vi "get-locking.vi"() -> (0 "error out":errorcluster, 3 "locking":u8)   [LabVIEW 2014]
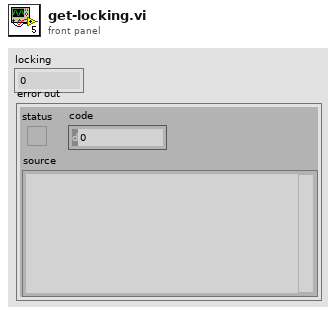
[diagram p1: front panel]
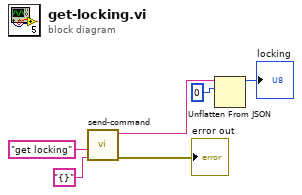
[diagram p0: block diagram]
diagram:
  n1 = call "send-command.vi"("parameters"="{}", "command"="get locking") -> ("error out"=→"error out":errorcluster, "output"=w3:string)  [unwired: 8 in]
  n2 = Unflatten From JSON(JSON string=w3, type and defaults=u8 0) -> (value=→"locking":u8)  [unwired: 5 in, 1 out]
